vi "trigier.vi"(7 "enum":T6(ring), 9 "manual save":bool, 10 "Virb Wave":waveform(dbl)[](array[waveform]), 11 "Task Info":T1={"Accele Task"=[], "Simulate"=FALSE, "采样率"={"AISampleRate"=10123, "CouplingType"=10000, "Butter"=1000}, "Trig"={"PreTrigCNT"=0, "TriggerMode"=enum."中间触发", "TriggerSource"=enum."软件触发", "ATRTriggerChannel"=enum."通道0", "TriggerDir"=enum."下降沿触发", "TrigLevelVolt"=0.0, "bAvailableTrig"=FALSE}, "clock"={"EN"=FALSE, "clocksource"=enum."内部时钟", "outclocksource"=enum."Trig0"}, "delay(S)"=0.0} {"采样率"."CouplingType" items=["直流耦合", "交流耦合"]}) -> (2 "triger?":bool, 3 "save?":bool)   [LabVIEW 2011]
uses:
  Ctrls/Task Info.ctl
  Ctrls/Sample Information.ctl
  Ctrls/Trig.ctl
  Ctrls/clock.ctl
  <vilib>/measure/macond.llb/FIR Filter for 1 Chan.vi
  <vilib>/Analysis/NI_AALBase.lvlib
  <vilib>/measure/NI_MAPro.lvlib
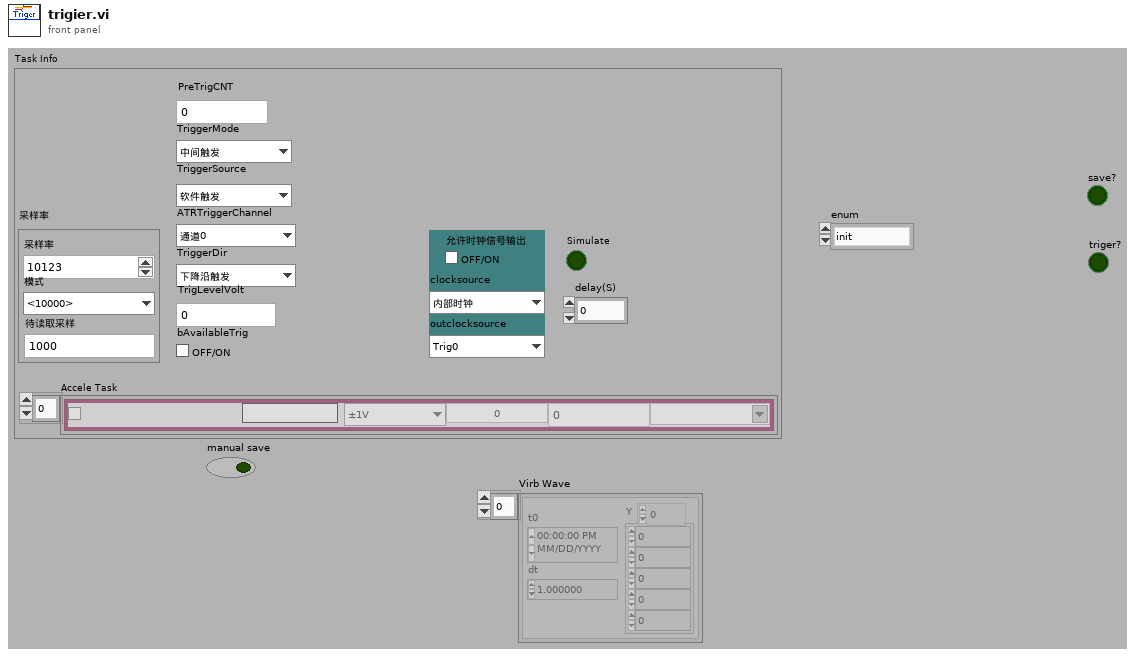
[diagram p1: front panel]
types:
  T1 = typedef "Task Info.ctl" = cluster{"Accele Task":T2[], "Simulate":bool, "采样率":T3, "Trig":T4, "clock":T5, "delay(S)":dbl}
  T2 = typedef "Acceleration Channel Config_Ctrls-某型振动实验台测试系统.ctl" = cluster{"Enable":bool, "Name":string, "range":enum16{"±1V", "±5V"}, "SensValue":dbl, "PhysicalName":string, "off":dbl, "Sensunits":string}
  T3 = typedef "Sample Information.ctl" = cluster{"AISampleRate":i32, "CouplingType":i32, "Butter":i32}
  T4 = typedef "Trig.ctl" = cluster{"PreTrigCNT":i32, "TriggerMode":enum16{"中间触发", "后触发", "预触发", "硬件延时触发"}, "TriggerSource":enum16{"软件触发", "DTR信号源", "ATR信号源", "Triger信号触发"}, "ATRTriggerChannel":enum16{"通道0", "通道1", "通道2", "通道3"}, "TriggerDir":enum16{"下降沿触发", "上升沿触发", "上下边没均触发"}, "TrigLevelVolt":sgl, "bAvailableTrig":bool}
  T5 = typedef "clock.ctl" = cluster{"EN":bool, "clocksource":enum16{"内部时钟", "外部时钟"}, "outclocksource":enum16{"Trig0", "Trig1", "Trig2", "Trig3", "Trig4", "Trig5", "Trig6", "Trig7", "PXI_STAR"}}
  T6 = enum16{"init", "trig", "save", "stop", "Default"}
  T7 = cluster{"index":i32, "delay":dbl, "threshold":dbl}
  T8 = cluster{"Topology":enum16{"Off", "FIR by Specification", "Equi-ripple FIR", "Windowed FIR"}, "Type":enum16{"Lowpass", "Highpass", "Bandpass", "Bandstop"}, "#Taps":i32, "Lower PB":dbl, "Upper PB":dbl, "Lower SB":dbl, "Upper SB":dbl}
  T9 = typedef "Enum File IO - FGV(V)_Ctrls-某型振动实验台测试系统.ctl" = enum16{"New", "Open", "Write Info", "Write Data", "Read Info", "Read Chan Names", "Read Data", "Close", "None"}
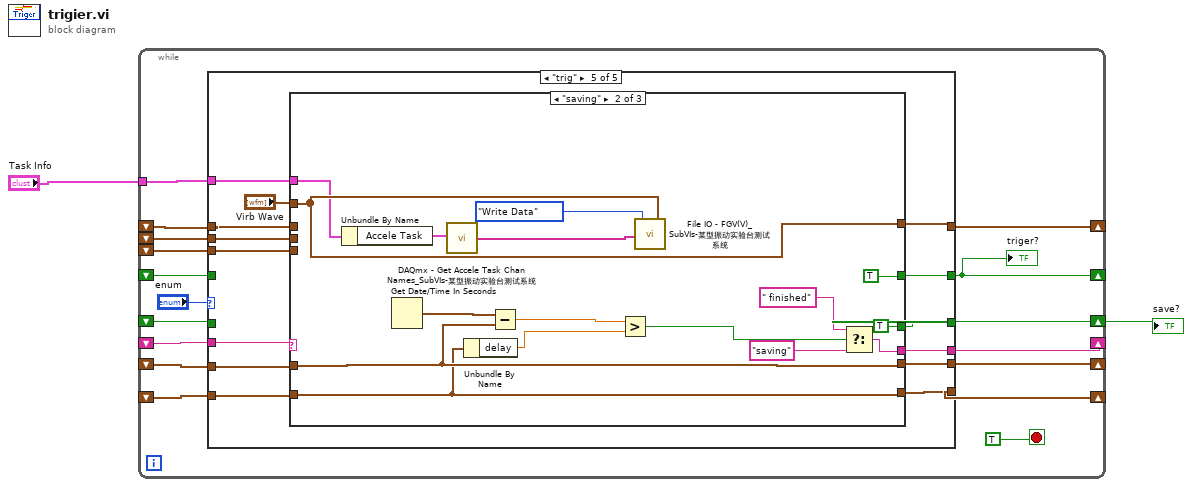
[diagram p0: block diagram]
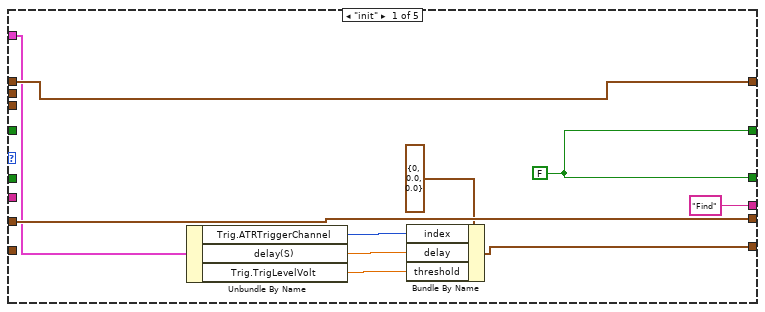
[diagram p2: hidden frame]
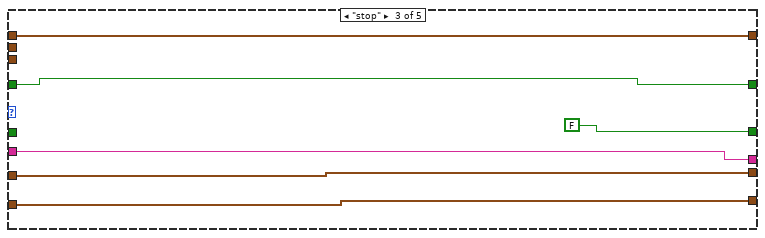
[diagram p4: hidden frame]
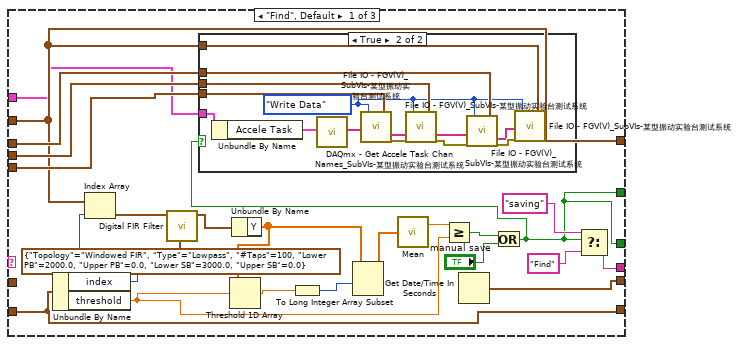
[diagram p6: hidden frame]
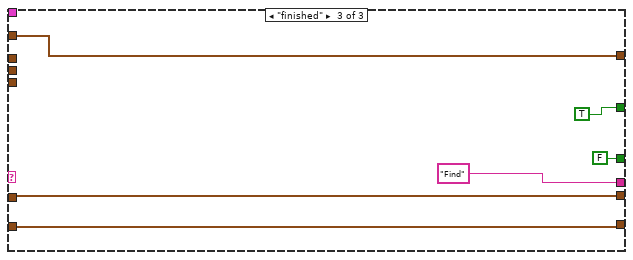
[diagram p8: hidden frame]
diagram:
  n1 = while {
    shift-right: [w12] -> w2
    shift-left: _ -> [w4]
    shift-right: [w17] -> _
    shift-left: _ -> [w16]
    shift-right: [w15] -> _
    shift-left: _ -> [w14]
    shift-right: [w13] -> _
    shift-left: _ -> [w5]
    shift-right: [w11] -> _
    shift-left: _ -> [w10]
    shift-left: _ -> [w9]
    shift-left: _ -> [w8]
    shift-right: [w7] -> _
    shift-left: _ -> [w6]
    tunnel: "Task Info" -> [w3]
    stop <- TRUE stop-if-true
    n2 = case shown="\"trig\"" "enum" {
      tunnel: [w23 w35 FALSE w47 w60] -> w12
      tunnel: w4 -> [_ w35 _ w47 _]
      tunnel: [w29 w34 w40 w46 w59] -> w17
      tunnel: w16 -> [w29 w34 w40 w46 w58]
      tunnel: [w27 w33 w39 w45 w56] -> w15
      tunnel: w14 -> [_ w33 w39 w45 w57]
      tunnel: [w23 w32 w38 w44 w49] -> w13
      tunnel: w5 -> [_ w32 w38 w44 _]
      tunnel: [w22 w31 w37 w43 w55] -> w11
      tunnel: w10 -> [w22 w31 w37 w43 w54]
      tunnel: w9 -> [_ _ _ _ w53]
      tunnel: w8 -> [_ _ _ _ w52]
      tunnel: ["Find" w30 w36 w42 w51] -> w7
      tunnel: w6 -> [_ w30 w36 w42 w50]
      tunnel: w3 -> [w20 _ _ _ w48]
      frame "init" {
        w23 = FALSE
        n3 = Unbundle By Name(w20) -> ("Trig.ATRTriggerChannel"=w26:enum16{"通道0", "通道1", "通道2", "通道3"}, "delay(S)"=w25:dbl, "Trig.TrigLevelVolt"=w24:sgl)
        n4 = Bundle By Name(cluster=T7 {"index"=0, "delay"=0.0, "threshold"=0.0} ("set"), "index"=w26, "delay"=w25, "threshold"=w24) -> (w27:T7)
      }
      frame "save" {
      }
      frame "stop" {
      }
      frame "Default", Default {
      }
      frame "trig" {
        n5 = case shown="\"saving\"" w50 {
          tunnel: "Virb Wave" -> [w70 w109 w117]
          tunnel: [w68 TRUE FALSE] -> w60
          tunnel: [w69 w113 w120] -> w59
          tunnel: w58 -> [_ w113 w120]
          tunnel: w57 -> [w79 w112 w119]
          tunnel: [w79 w112 w119] -> w56
          tunnel: [w68 TRUE TRUE] -> w49
          tunnel: [w70 w109 w117] -> w55
          tunnel: w54 -> [w78 _ _]
          tunnel: w53 -> [w77 _ _]
          tunnel: w52 -> [w76 _ _]
          tunnel: [w73 w107 "Find" ("f")] -> w51
          tunnel: w48 -> [w62 w104 _]
          frame "Find", Default {
            n6 = Unbundle By Name(w79) -> ("index"=w80:i32, "threshold"=w67:dbl)
            n7 = Index Array(array=w70, index=w80) -> (element=w65:waveform(dbl))
            n8 = call-poly <vilib>:"Digital FIR Filter.vi"("FIR filter specifications"=T8 {"Topology"=enum."Windowed FIR", "Type"=enum."Lowpass", "#Taps"=100, "Lower PB"=2000.0, "Upper PB"=0.0, "Lower SB"=3000.0, "Upper SB"=0.0}, "signal in"=w65) -> ("signal out"=w64:waveform(dbl))  [unwired: 3 in, 6 out]
            n9 = Unbundle By Name(w64) -> ("Y"=w66:dbl[])
            n10 = Threshold 1D Array(2:w67, 3:w66) -> (0:w84:dbl)  [unwired: 1 out]
            n11 = To Long Integer(number=w84) -> (32bit integer=w83:i32)
            n12 = Array Subset(array=w66, index=w83) -> (w81:dbl[])  [unwired: 1 in]
            n13 = call <vilib>:"Mean.vi"("X"=w81) -> ("mean"=w82:dbl)  [unwired: 1 out]
            n14 = Greater Or Equal?(x=w82, y=w67) -> (x >= y?=w71:bool)
            n15 = Get Date/Time In Seconds() -> (seconds since 1Jan1904=w69:timestamp)
            n16 = Or(x=w71, y="manual save") -> (x .or. y?=w68:bool)
            n17 = case shown="True" w68 {
              tunnel: w78 -> [_ w98]
              tunnel: w77 -> [_ w97]
              tunnel: w76 -> [_ w96]
              tunnel: w70 -> [_ w91]
              tunnel: w62 -> [_ w90]
              frame False {
              }
              frame True {
                w95 = Enum_File_IO_-_FGV(V)_Ctrls-某型振动实验台测试系统."Write Data" ("Operation")
                n18 = Unbundle By Name(w90) -> ("Accele Task"=w89:T2[])
                n19 = call "DAQmx - Get Accele Task Chan Names_SubVIs-某型振动实验台测试系统.vi"("Accele Task"=w89) -> ("Chan Names"=w88:string[])
                n20 = call "File IO - FGV(V)_SubVIs-某型振动实验台测试系统.vi"("Vibration Channel Name Input"=w88, "Operation"=w95, "Vibration Waveform"=w96) -> ("Vibration Chan Names Out"=w87:string[], "error out"=w94:errorcluster)  [unwired: 7 in, 8 out]
                n21 = call "File IO - FGV(V)_SubVIs-某型振动实验台测试系统.vi"("Vibration Channel Name Input"=w87, "error in"=w94, "Operation"=w95, "Vibration Waveform"=w97) -> ("Vibration Chan Names Out"=w86:string[], "error out"=w93:errorcluster)  [unwired: 6 in, 8 out]
                n22 = call "File IO - FGV(V)_SubVIs-某型振动实验台测试系统.vi"("Vibration Channel Name Input"=w86, "error in"=w93, "Operation"=w95, "Vibration Waveform"=w98) -> ("Vibration Chan Names Out"=w85:string[], "error out"=w92:errorcluster)  [unwired: 6 in, 8 out]
                n23 = call "File IO - FGV(V)_SubVIs-某型振动实验台测试系统.vi"("Vibration Channel Name Input"=w85, "error in"=w92, "Operation"=w95, "Vibration Waveform"=w91) -> ()  [unwired: 6 in, 10 out]
              }
            }
            n24 = Select(t="saving", s=w68, f="Find") -> (s? t:f=w73:string)
          }
          frame "saving" {
            n25 = Unbundle By Name(w104) -> ("Accele Task"=w103:T2[])
            n26 = Get Date/Time In Seconds() -> (seconds since 1Jan1904=w114:timestamp)
            n27 = call "DAQmx - Get Accele Task Chan Names_SubVIs-某型振动实验台测试系统.vi"("Accele Task"=w103) -> ("Chan Names"=w102:string[])
            n28 = Unbundle By Name(w112) -> ("delay"=w100:dbl)
            n29 = Subtract(x=w114, y=w113) -> (x-y=w101:dbl)
            n30 = Greater?(x=w101, y=w100) -> (0:w99:bool)
            n31 = call "File IO - FGV(V)_SubVIs-某型振动实验台测试系统.vi"("Vibration Channel Name Input"=w102, "Operation"=Enum_File_IO_-_FGV(V)_Ctrls-某型振动实验台测试系统."Write Data", "Vibration Waveform"=w109) -> ()  [unwired: 7 in, 10 out]
            n32 = Select(t=" finished" ("f"), s=w99, f="saving") -> (s? t:f=w107:string)
          }
          frame "finished" {
          }
        }
      }
    }
    "triger?" <- w13
  }
  "save?" <- w2
